vi "bioprinterv1.2.vi"() -> ()   [LabVIEW 2020]
uses:
  <vilib>/MakerHub/LINX/Public/Peripherals/Digital/Digital Write 1 Chan.vi
  <vilib>/MakerHub/LINX/Public/Peripherals/Digital/Digital Write N Chans.vi
  <vilib>/MakerHub/LINX/Private/Local IO/LinxDigitalWrite.vi
  <vilib>/MakerHub/LINX/Public/Utilities/Check Channel.vi
  <vilib>/MakerHub/LINX/Public/Utilities/Open Serial.vi
  <vilib>/MakerHub/LINX/Private/Utilties/Generate Error.vi
  <vilib>/MakerHub/LINX/LMH-LINX.lvlib
panel:
  in  "Feed - Suction":bool
  in  "Volumetric Flow Rate(mm^3/sn)":dbl
  in  "Emergency stop? (T)":bool
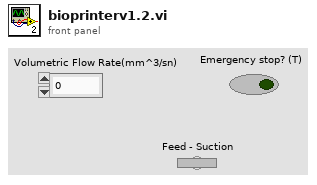
[diagram p1: front panel]
types:
  T1 = typedef "LMH-LINX.lvlib/LINX Ref.ctl" = cluster{"IO":T2, "Interface":T3, "LINX Device Config":T4}
  T2 = typedef "LMH-LINX.lvlib/Platform.ctl" = enum16{"Remote", "Local"}
  T3 = typedef "LMH-LINX.lvlib/Interface.ctl" = enum16{"Serial", "TCP"}
  T4 = typedef "LMH-LINX.lvlib/Device.lvlib/LINX Device Config.ctl" = cluster{"Interface":T3, "COM Port":refnum<visa-resource-name>, "TCP Configuration":T5, "Device Family":u8, "Device ID":u8, "Device Name":string, "TCP Ref":refnum<k5>, "Channels":T6}
  T5 = typedef "LMH-LINX.lvlib/Device.lvlib/TCP Config.ctl" = cluster{"IP Address":string, "Port":u16}
  T6 = typedef "LMH-LINX.lvlib/Channels.ctl" = cluster{"DI":u8[], "DO":u8[], "AI":u8[], "AO":u8[], "PWM":u8[], "QE":u8[], "UART":u8[], "I2C 2":u8[], "SPI":u8[], "CAN":u8[], "Servo":u8[], "AI Ref (V)":dbl, "AI Resolution (Bits)":u8, "AO Ref (V)":dbl, "AO Resolution (Bits)":u8}
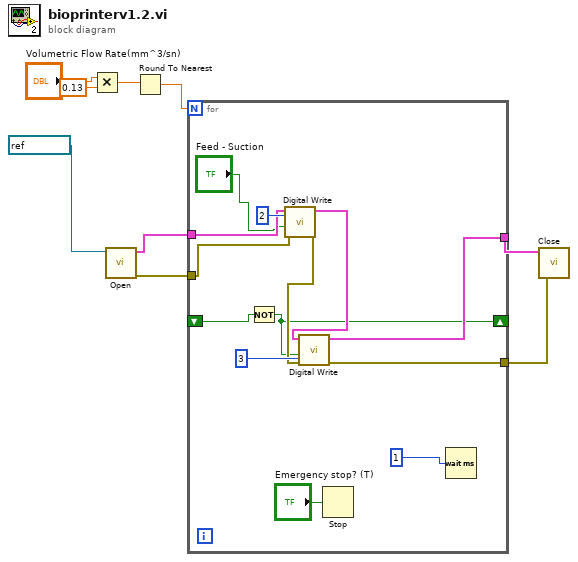
[diagram p0: block diagram]
diagram:
  n1 = Multiply(x="Volumetric Flow Rate(mm^3/sn)", y=0.13) -> (x*y=w2:dbl)
  n2 = call-poly <vilib>:"Open.vi"("Serial Port"=refnum<visa-resource-name> "COM6") -> ("Error Out"=w6:errorcluster, "LINX Resource"=w8:T1)  [unwired: 8 in, 1 out]
  n3 = Round To Nearest(number=w2) -> (nearest integer value=w1:dbl)
  n4 = for {
    N: w1 -> [_]
    tunnel: w8 -> [w20]
    tunnel: [w18] -> w7
    tunnel: w6 -> [w17]
    tunnel: [w15] -> w5
    shift-right: [w13] -> _
    shift-left: _ -> [w14]
    n5 = Not(x=w14) -> (.not. x?=w13:bool)
    n6 = call-poly <vilib>:"Digital Write.vi"("Error In"=w17, "Output Value"="Feed - Suction", "DO Channel"=u8 2, "LINX Resource"=w20) -> ("Error Out"=w16:errorcluster, "LINX Resource"=w19:T1)  [unwired: 6 in]
    n7 = call-poly <vilib>:"Digital Write.vi"("Error In"=w16, "Output Value"=w13, "DO Channel"=u8 3, "LINX Resource"=w19) -> ("Error Out"=w15:errorcluster, "LINX Resource"=w18:T1)  [unwired: 6 in]
    n8 = Stop(stop? (T)="Emergency stop? (T)") -> ()
    n9 = Wait (ms)(milliseconds to wait=u32 1 ("millisecond timer value")) -> ()  [unwired: 1 out]
  }
  n10 = call <vilib>:"Close.vi"("Error In"=w5, "LINX Resource"=w7) -> ()  [unwired: 9 in, 1 out]
